vi "Operate_on_EEPROM.vi"(6 "Operation":enum16{"Write", "Read"}(ring), 7 "EEPROM Addresses":u8(ring) items=["I2C Slave Address", "Magnetometer X Offset MSB", "Magnetometer X Offset LSB", "Magnetometer Y Offset MSB", "Magnetometer Y Offset LSB", "Measurement Time Delay", "Number of Summed Measurements", "Software Version Number", "Operation Mode Byte"], 8 "error in (no error)":errorcluster, 9 "I2C Channel":u8, 10 "Data":u8, 11 "LINX Resource In":T1) -> (0 "error out":errorcluster, 2 "Data Out":u8[](array[numeric]), 3 "LINX Resource Out":T1)   [LabVIEW 2014, in "LMH-LINX.lvlib" / "HMC6352.lvlib"]
uses:
  <vilib>/MakerHub/LINX/Public/Sensors/Orientation/Compass/HMC6352/HMC6352.lvlib
  <vilib>/MakerHub/LINX/Private/Type Defs/LINX Ref.ctl
  <vilib>/MakerHub/LINX/Private/Type Defs/Platform.ctl
  <vilib>/MakerHub/LINX/Private/Type Defs/Interface.ctl
  <vilib>/MakerHub/LINX/Private/Device/Type Defs/LINX Device Config.ctl
  <vilib>/MakerHub/LINX/Private/Device/Type Defs/TCP Config.ctl
  <vilib>/MakerHub/LINX/Private/Device/Type Defs/Channels.ctl
  <vilib>/MakerHub/LINX/Private/Local IO/LinxI2cWrite.vi
  <vilib>/MakerHub/LINX/Public/Utilities/Check Channel.vi
  <vilib>/MakerHub/LINX/Private/Utilties/Generate Error.vi
  <vilib>/MakerHub/LINX/LMH-LINX.lvlib
  <vilib>/MakerHub/LINX/Private/Device/Device.lvlib
panel:
  # "INPUTS"
  # "OUTPUTS"
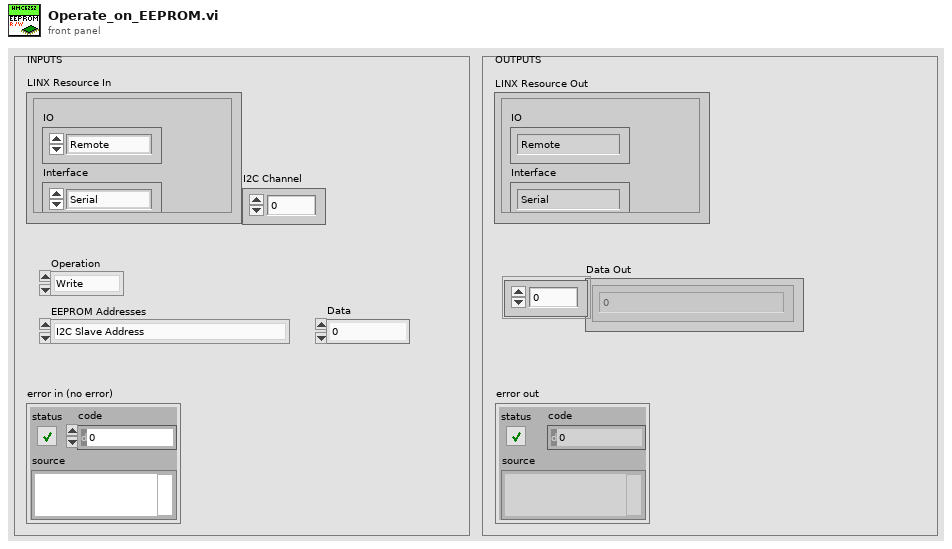
[diagram p1: front panel]
types:
  T1 = typedef "LMH-LINX.lvlib/LINX Ref.ctl" = cluster{"IO":T2, "Interface":T3, "LINX Device Config":T4}
  T2 = typedef "LMH-LINX.lvlib/Platform.ctl" = enum16{"Remote", "Local"}
  T3 = typedef "LMH-LINX.lvlib/Interface.ctl" = enum16{"Serial", "TCP"}
  T4 = typedef "LMH-LINX.lvlib/Device.lvlib/LINX Device Config.ctl" = cluster{"Interface":T3, "COM Port":refnum<visa-resource-name>, "TCP Configuration":T5, "Device Family":u8, "Device ID":u8, "Device Name":string, "TCP Ref":refnum<k5>, "Channels":T6}
  T5 = typedef "LMH-LINX.lvlib/Device.lvlib/TCP Config.ctl" = cluster{"IP Address":string, "Port":u16}
  T6 = typedef "LMH-LINX.lvlib/Channels.ctl" = cluster{"DI":u8[], "DO":u8[], "AI":u8[], "AO":u8[], "PWM":u8[], "QE":u8[], "UART":u8[], "I2C 2":u8[], "SPI":u8[], "CAN":u8[], "Servo":u8[], "AI Ref (V)":dbl, "AI Resolution (Bits)":u8, "AO Ref (V)":dbl, "AO Resolution (Bits)":u8}
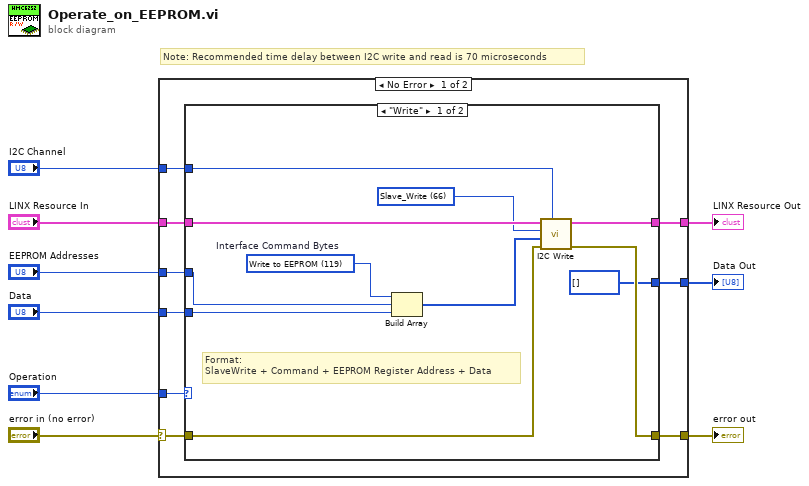
[diagram p0: block diagram]
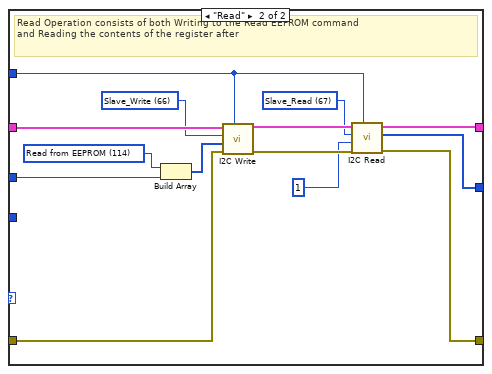
[diagram p2: hidden frame]
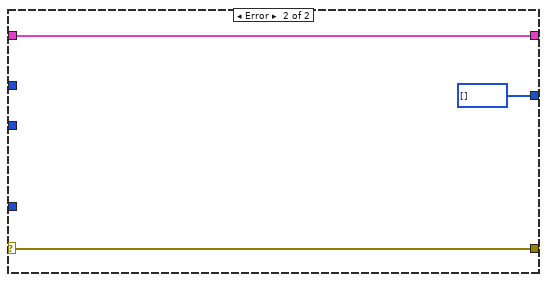
[diagram p3: hidden frame]
diagram:
  # "Note: Recommended time delay between I2C write and read is 70 microseconds"
  n1 = case shown="No Error" "error in (no error)" {
    selector: "error in (no error)" -> [w13 w46]
    tunnel: [w11 w46] -> w8
    tunnel: "LINX Resource In" -> [w17 w45]
    tunnel: "Operation" -> [w18 _]
    tunnel: "I2C Channel" -> [w16 _]
    tunnel: "Data" -> [w15 _]
    tunnel: "EEPROM Addresses" -> [w14 _]
    tunnel: [w12 w45] -> w2
    tunnel: [w10 u8[] [] ("Data")] -> w1
    frame No Error {
      n2 = case shown="\"Write\"" w18 {
        tunnel: w17 -> [w29 w43]
        tunnel: w16 -> [w28 w35]
        tunnel: w15 -> [w19 _]
        tunnel: w14 -> [w20 w40]
        tunnel: w13 -> [w24 w42]
        tunnel: [w23 w34] -> w12
        tunnel: [w22 w30] -> w11
        tunnel: [u8[] [] ("Data") w33] -> w10
        frame "Write" {
          w26 = u8 119 items=["Write to EEPROM"=119, "Read from EEPROM"=114, "Write to RAM Register"=71, "Read from RAM Register"=103, "Enter Sleep Mode"=83, "Exit Sleep Mode"=87, "Update Bridge Offsets (Set/Reset)"=79, "Enter User Calibration Mode"=67, "Exit User Calibration Mode"=69, "Save Operation Mode to EEPROM"=76, "J_Who_am_i"=117, "Get Data/Calculate New Heading"=65]  # Interface Command Bytes
          w27 = u8 66 items=["Slave_Write"=66, "Slave_Read"=67, "J_Test"=104] ("HMC6352 Slave Address")
          # "Format:\nSlaveWrite + Command + EEPROM Register Address + Data"
          n3 = Build Array(w26, w20, w19) -> (w25:u8[])
          n4 = call <vilib>:"I2C Write.vi"("I2C Channel"=w28, "Error In"=w24, "Data"=w25, "I2C Slave Address (0)"=w27, "LINX Resource"=w29) -> ("Error Out"=w22:errorcluster, "LINX Resource"=w23:T1)  [unwired: 5 in]
        }
        frame "Read" {
          w36 = u8 67 items=["Slave_Write"=66, "Slave_Read"=67] ("HMC6352 Slave Address")
          w41 = u8 66 items=["Slave_Write"=66, "Slave_Read"=67] ("HMC6352 Slave Address")
          w32 = u8 114 items=["Write to EEPROM"=119, "Read from EEPROM"=114, "Write to RAM Register"=71, "Read from RAM Register"=103, "Enter Sleep Mode"=83, "Exit Sleep Mode"=87, "Update Bridge Offsets (Set/Reset)"=79, "Enter User Calibration Mode"=67, "Exit User Calibration Mode"=69, "Save Operation Mode to EEPROM"=76, "Get Data/Calculate New Heading"=65] ("Interface Command Bytes")
          # "Read Operation consists of both Writing to the Read EEPROM command\nand Reading the contents of the register after"
          n5 = Build Array(w32, w40) -> (w39:u8[])
          n6 = call <vilib>:"I2C Write.vi"("I2C Channel"=w35, "Error In"=w42, "Data"=w39, "I2C Slave Address (0)"=w41, "LINX Resource"=w43) -> ("Error Out"=w37:errorcluster, "LINX Resource"=w38:T1)  [unwired: 5 in]
          n7 = call <vilib>:"I2C Read.vi"("I2C Channel"=w35, "Error In"=w37, "Bytes To Read"=u8 1, "I2C Slave Address (0)"=w36, "LINX Resource"=w38) -> ("Error Out"=w30:errorcluster, "Data"=w33:u8[], "LINX Resource"=w34:T1)  [unwired: 4 in]
        }
      }
    }
    frame Error {
    }
  }
  "LINX Resource Out" <- w2
  "error out" <- w8
  "Data Out" <- w1
